vi "Get_Ch_data_from_file.vi"(0 "Filename":path, 9 "Channel names":string[](array[string]), 11 "Start of read offset (chars.: 0)":i32, 12 "Averaging Time(s)":dbl=5.0) -> (4 "exists?":bool, 6 "File Channels":string[](array[string]), 10 "Times":dbl[](array[numeric]) format="%.2f", 15 "Ch Data":dbl[][](array[numeric]) format="%.2f")   [LabVIEW 2010]
uses:
  <vilib>/Analysis/NI_AALBase.lvlib
panel:
  out "Time difference":dbl format="%.2f"
  in  "stop":bool
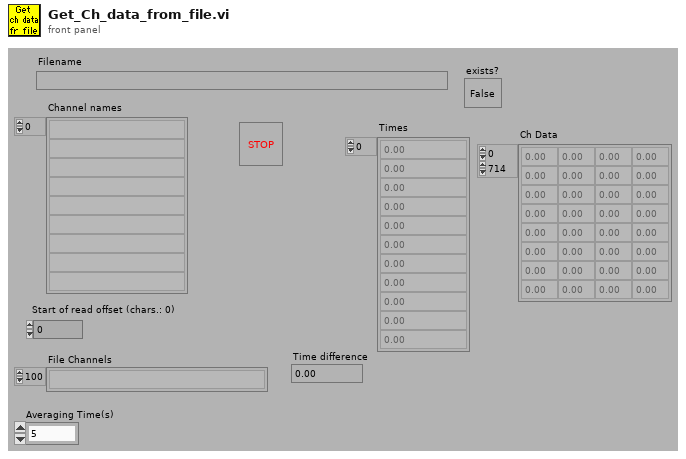
[diagram p1: front panel]
types:
  T1 = cluster{"second":i32, "minute":i32, "hour":i32, "day of month":i32, "month":i32, "year":i32, "day of week":i32, "day of year":i32, "is DST":i32}
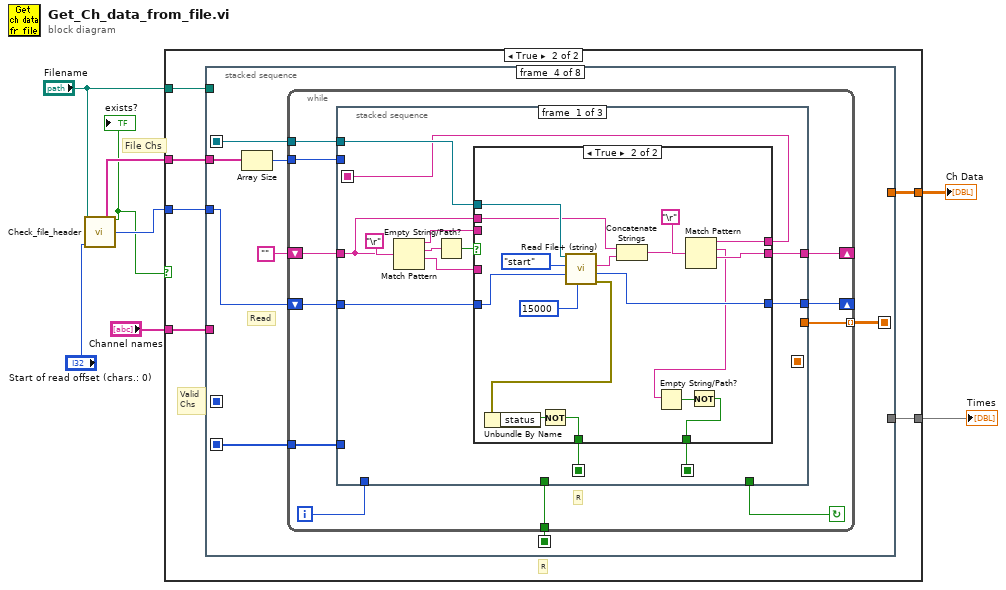
[diagram p0: block diagram]
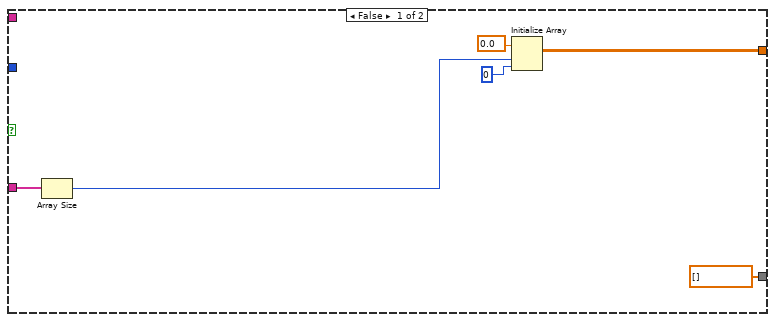
[diagram p2: hidden frame]
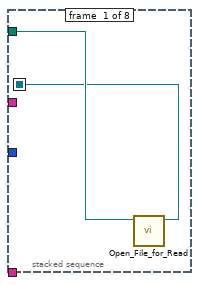
[diagram p3: hidden frame]
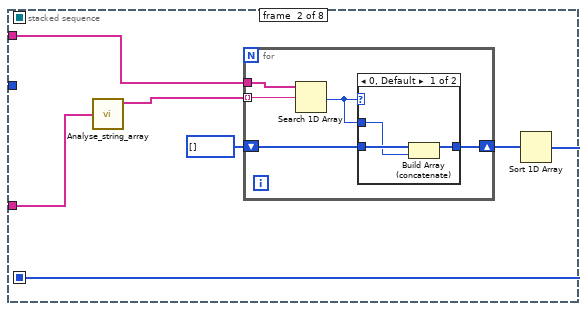
[diagram p4: hidden frame]
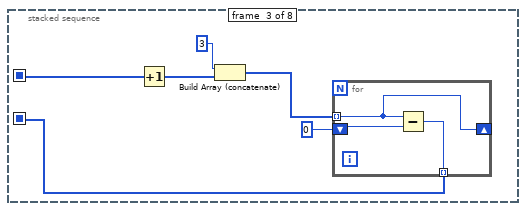
[diagram p6: hidden frame]
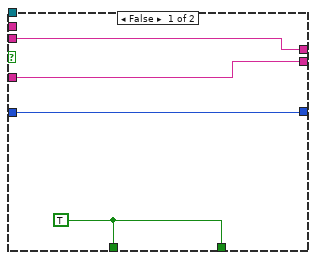
[diagram p7: hidden frame]
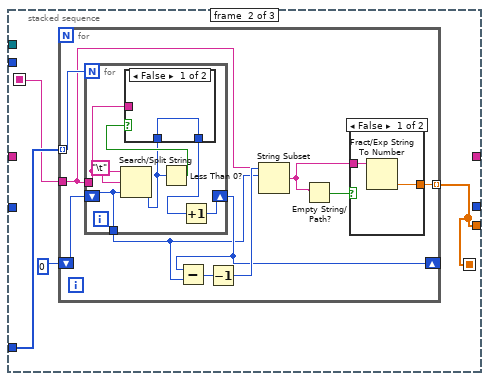
[diagram p8: hidden frame]
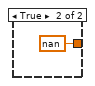
[diagram p9: hidden frame]
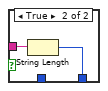
[diagram p10: hidden frame]
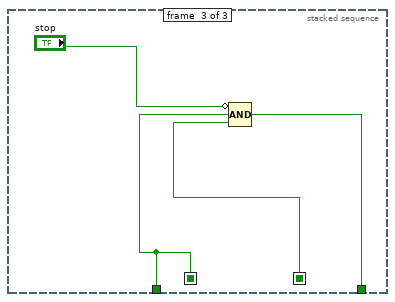
[diagram p11: hidden frame]
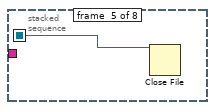
[diagram p12: hidden frame]
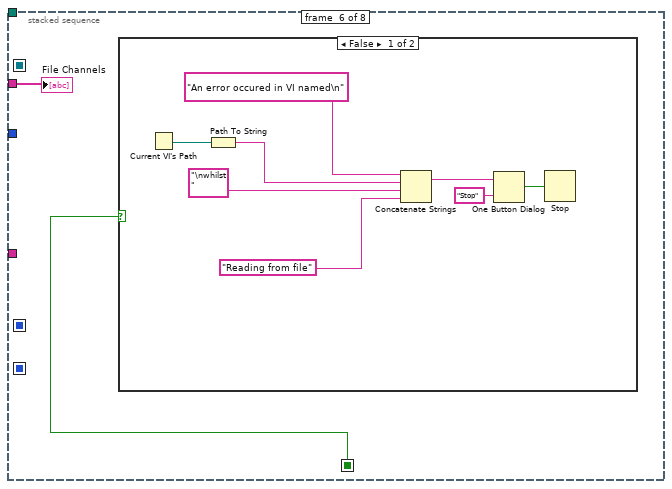
[diagram p13: hidden frame]
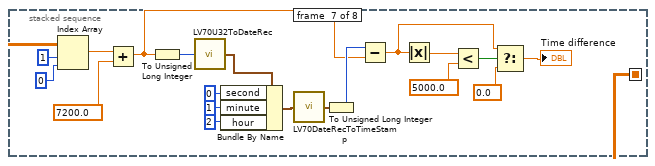
[diagram p15: hidden frame]
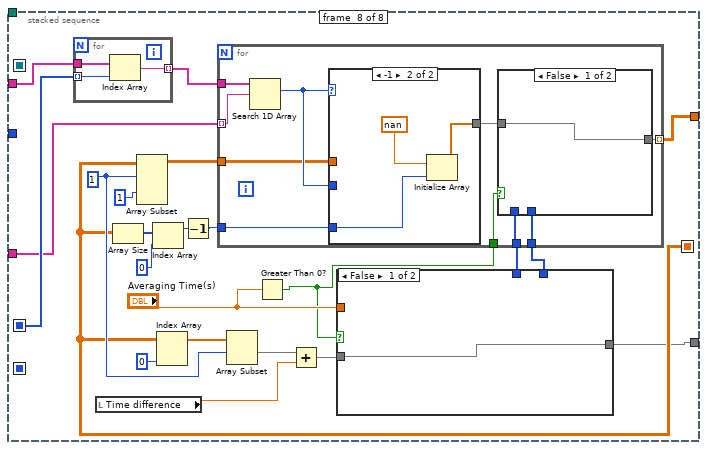
[diagram p16: hidden frame]
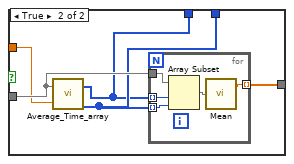
[diagram p17: hidden frame]
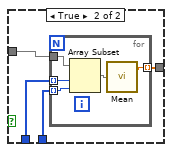
[diagram p18: hidden frame]
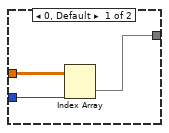
[diagram p19: hidden frame]
diagram:
  # "File Chs"
  n1 = call "Check_file_header.vi"("Filename"="Filename", "Start of read offset (chars.: 0)"="Start of read offset (chars.: 0)") -> ("File Channels"=w7:string[], "exists?"=w4:bool, "Start of data (bytes)"=w8:i32)  [unwired: 2 in, 9 out]
  "exists?" <- w4
  n2 = case shown="True" w4 {
    tunnel: w8 -> [_ w19]
    tunnel: w7 -> [_ w18]
    tunnel: "Filename" -> [_ w20]
    tunnel: [w9 w16] -> w3
    tunnel: [dbl[] [] w15] -> w2
    tunnel: "Channel names" -> [w11 w17]
    frame False {
      n3 = Array Size(array=w11) -> (size(s)=w10:i32)
      n4 = Initialize Array(0.0, w10, 0 ("Dimension Size")) -> (w9:dbl[][])
    }
    frame True {
      # "Valid\nChs"
      # "R"
      n5 = stacked-sequence {
        seq-local: [w21 _ _ _ _ _ _ _] -> [_ _ _ w53 w131 _ _ _]
        seq-local: [_ _ _ w50 _ _ _ _] -> [_ _ _ _ _ w133 _ _]
        seq-local: [_ _ _ w48 _ _ _ _] -> [_ _ _ _ _ _ w159 w173]
        seq-local: [_ _ w41 _ _ _ _ _] -> [_ _ _ w47 _ _ _ _]
        seq-local: [_ w25 _ _ _ _ _ _] -> [_ _ w39 _ _ _ _ w178]
        tunnel: w20 -> [w22 _ _ _ _ _ _ _]
        tunnel: w19 -> [_ _ _ w52 _ _ _ _]
        tunnel: w18 -> [_ w28 _ w49 _ w132 _ w177]
        tunnel: w17 -> [_ w24 _ _ _ _ _ w176]
        tunnel: [_ _ _ _ _ _ _ w169] -> w16
        tunnel: [_ _ _ _ _ _ _ w166] -> w15
        frame #0 {
          n6 = call "Open_File_for_Read.vi"("file path"=w22) -> ("refnum"=w21:refnum<file>)  [unwired: 1 in, 9 out]
        }
        frame #1 {
          n7 = call "Analyse_string_array.vi"("String array"=w24) -> ("Unique strings"=w23:string[])  [unwired: 2 out]
          n8 = for {
            tunnel: w28 -> [w33]
            tunnel: w23 -> [w32] mode=indexing
            shift-right: [w30] -> w26
            shift-left: i32[] [] -> [w31]
            n9 = Search 1D Array(1D array=w33, element=w32) -> (index of element=w29:i32)  [unwired: 1 out]
            n10 = case shown="0, Default" w29 {
              tunnel: w31 -> [w36 w37]
              tunnel: [w34 w37] -> w30
              tunnel: w29 -> [w35 _]
              frame 0, Default {
                n11 = Build Array (concatenate)(w36, w35) -> (w34:i32[])
              }
              frame -1 {
              }
            }
          }
          n12 = Sort 1D Array(array=w26) -> (sorted array=w25:i32[])
        }
        frame #2 {
          n13 = Increment(x=w39) -> (x+1=w38:i32[])
          n14 = Build Array (concatenate)(3 ("t"), w38) -> (w40:i32[])
          n15 = for {
            shift-right: [w45] -> _
            shift-left: 0 -> [w46]
            tunnel: w40 -> [w45] mode=indexing
            tunnel: [w44] -> w41 mode=indexing
            n16 = Subtract(x=w45, y=w46) -> (x-y=w44:i32)
          }
        }
        frame #3 {
          # "Read"
          n17 = Array Size(array=w49) -> (size(s)=w51:i32)
          n18 = while {
            tunnel: w47 -> [w56]
            tunnel: [w58] -> w48 mode=indexing
            tunnel: [w59] -> w50
            tunnel: w51 -> [w60]
            tunnel: w53 -> [w62]
            shift-left: w52 -> [w64]
            shift-right: [w63] -> _
            shift-left: "" -> [w65]
            shift-right: [w61] -> _
            i -> [w57]
            stop <- w55 continue-if-true
            # "R"
            n19 = stacked-sequence {
              seq-local: [w67 _ _] -> [_ w101 _]
              seq-local: [w68 _ _] -> [_ _ w127]
              seq-local: [w69 _ _] -> [_ _ w128]
              seq-local: [_ w100 _] -> [_ _ _]
              tunnel: w65 -> [w72 _ _]
              tunnel: w64 -> [w75 _ _]
              tunnel: [w74 _ _] -> w63
              tunnel: w62 -> [w73 _ _]
              tunnel: [w71 _ _] -> w61
              tunnel: w60 -> [_ _ _]
              tunnel: [_ _ w129] -> w55
              tunnel: [_ _ w128] -> w59
              tunnel: [_ w100 _] -> w58
              tunnel: w57 -> [_ _ _]
              tunnel: w56 -> [_ w103 _]
              frame #0 {
                n20 = Match Pattern(string=w72, regular expression="\r") -> (before substring=w66:string, match substring=w77:string, after substring=w70:string)  [unwired: 2 out]
                n21 = Empty String/Path?(string/path=w77) -> (empty?=w76:bool)
                n22 = case shown="True" w76 {
                  tunnel: w75 -> [w82 w98]
                  tunnel: [w82 w96] -> w74
                  tunnel: w73 -> [_ w95]
                  tunnel: w72 -> [_ w93]
                  tunnel: [w81 w90] -> w71
                  tunnel: w70 -> [w81 _]
                  tunnel: [w80 w86] -> w69
                  tunnel: [w80 w84] -> w68
                  tunnel: [w79 w83] -> w67
                  tunnel: w66 -> [w79 _]
                  frame False {
                    w80 = TRUE
                  }
                  frame True {
                    n23 = call <vilib>:"Read File+ (string).vi"("count"=15000, "pos offset (bytes:0)"=w98, "pos mode (rel. to current:2)"=enum16{"start", "end", "current"}."start", "refnum"=w95) -> ("error out"=w88:errorcluster, "mark after read (bytes)"=w96:i32, "string"=w94:string)  [unwired: 1 in, 4 out]
                    n24 = Unbundle By Name(w88) -> ("status"=w87:bool)
                    n25 = Not(x=w87) -> (.not. x?=w86:bool)
                    n26 = Concatenate Strings(w93, w94) -> (w91:string)
                    n27 = Match Pattern(string=w91, regular expression="\r") -> (before substring=w83:string, match substring=w89:string, after substring=w90:string)  [unwired: 2 out]
                    n28 = Empty String/Path?(string/path=w89) -> (empty?=w85:bool)
                    n29 = Not(x=w85) -> (.not. x?=w84:bool)
                  }
                }
              }
              frame #1 {
                n30 = for {
                  tunnel: w103 -> [w113] mode=indexing
                  tunnel: [w111] -> w100 mode=indexing
                  shift-right: [w105] -> _
                  shift-left: 0 -> [w110]
                  tunnel: w101 -> [w106]
                  n31 = for {
                    N: w113 -> [_]
                    shift-right: [w121] -> w105
                    shift-left: w110 -> [w122]
                    tunnel: w106 -> [w119]
                    tunnel: [w122] -> w104
                    n32 = Search/Split String(string=w119, search string/char (-)="\t", offset (0)=w122) -> (offset of match=w117:i32)  [unwired: 2 out]
                    n33 = Less Than 0?(x=w117) -> (x < 0?=w120:bool)
                    n34 = case shown="False" w120 {
                      tunnel: w119 -> [_ w126]
                      tunnel: [w124 w125] -> w118
                      tunnel: w117 -> [w124 _]
                      frame False {
                      }
                      frame True {
                        n35 = String Length(string=w126) -> (length=w125:i32)
                      }
                    }
                    n36 = Increment(x=w118) -> (x+1=w121:i32)
                  }
                  n37 = Subtract(x=w105, y=w104) -> (x-y=w109:i32)
                  n38 = Decrement(x=w109) -> (x-1=w108:i32)
                  n39 = String Subset(string=w106, offset (0)=w104, length (rest)=w108) -> (substring=w107:string)
                  n40 = Empty String/Path?(string/path=w107) -> (empty?=w112:bool)
                  n41 = case shown="False" w112 {
                    tunnel: w107 -> [w115 _]
                    tunnel: [w114 nan] -> w111
                    frame False {
                      n42 = Fract/Exp String To Number(string=w115) -> (number=w114:dbl)  [unwired: 4 out]
                    }
                    frame True {
                    }
                  }
                }
              }
              frame #2 {
                n43 = Compound Arithmetic op=AND(invert "stop", w128, w127) -> (w129:bool)
              }
            }
          }
        }
        frame #4 {
          n44 = Close File(refnum=w131) -> ()  [unwired: 1 in, 2 out]
        }
        frame #5 {
          n45 = case shown="False" w133 {
            frame False {
              n46 = Current VI's Path() -> (path=w134:path)
              n47 = Path To String(path=w134) -> (string=w140:string)
              n48 = Concatenate Strings("An error occured in VI named\n", w140, "\nwhilst ", "Reading from file") -> (w138:string)
              n49 = One Button Dialog(message=w138, button name ("OK")="Stop") -> (true=w136:bool)
              n50 = Stop(stop? (T)=w136) -> ()
            }
            frame True {
            }
          }
          "File Channels" <- w132
        }
        frame #6 {
          n51 = Index Array(array=w159, index (row)=1 ("Index"), index (col)=0 ("Index")) -> (element=w146:dbl)
          n52 = Add(x=w146, y=7200.0) -> (x+y=w143:dbl)
          n53 = To Unsigned Long Integer(number=w143) -> (unsigned 32bit integer=w153:u32)
          n54 = call <vilib>:"LV70U32ToDateRec.vi"("Time"=w153) -> ("date time rec"=w158:T1)
          n55 = Bundle By Name(cluster=w158, "second"=0 ("Bundle Element"), "minute"=1 ("Bundle Element"), "hour"=2 ("Bundle Element")) -> (w154:T1)
          n56 = call <vilib>:"LV70DateRecToTimeStamp.vi"("date time rec"=w154) -> ("Time Stamp"=w142:timestamp)
          n57 = To Unsigned Long Integer(number=w142) -> (unsigned 32bit integer=w144:u32)
          n58 = Subtract(x=w144, y=w143) -> (x-y=w148:dbl)
          n59 = Absolute Value(x=w148) -> (abs(x)=w152:dbl)
          n60 = Less?(x=w152, y=5000.0) -> (x < y?=w150:bool)
          n61 = Select(t=w148, s=w150, f=0.0) -> (s? t:f=→"Time difference":dbl)
        }
        frame #7 {
          w181 = 1
          n62 = for {
            tunnel: w178 -> [w198] mode=indexing
            tunnel: w177 -> [w197]
            tunnel: [w196] -> w175 mode=indexing
            n63 = Index Array(array=w197, index=w198) -> (element=w196:string)
          }
          n64 = local read "Time difference"() -> (w179:dbl)
          n65 = Array Size(array=w173) -> (size(s)=w172:i32[])
          n66 = Array Subset(array=w173, index (row)=w181, index (col)=1) -> (w174:dbl[][])  [unwired: 2 in]
          n67 = Index Array(array=w172, index=0 ("Index")) -> (element=w170:i32)
          n68 = Index Array(array=w173, index (col)=0) -> (element=w182:dbl[])  [unwired: 1 in]
          n69 = Decrement(x=w170) -> (x-1=w168:i32)
          n70 = Array Subset(array=w182, index=w181) -> (w180:dbl[])  [unwired: 1 in]
          n71 = Greater Than 0?(x="Averaging Time(s)") -> (x > 0?=w162:bool)
          n72 = Add(x=w180, y=w179) -> (x+y=w167:dbl[])
          n73 = case shown="False" w162 {
            tunnel: w167 -> [w185 w190]
            tunnel: [w185 w189] -> w166
            tunnel: [_ w186] -> w165
            tunnel: [_ w188] -> w164
            tunnel: "Averaging Time(s)" -> [_ w187]
            frame False {
            }
            frame True {
              n74 = call "Average_Time_array.vi"("Average TIme (seconds)"=w187, "Centre Time in Seconds"=w190) -> ("Length"=w188:i32[], "Start"=w186:i32[])
              n75 = for {
                tunnel: w190 -> [w195]
                tunnel: w186 -> [w194] mode=indexing
                tunnel: w188 -> [w193] mode=indexing
                tunnel: [w191] -> w189 mode=indexing
                n76 = Array Subset(array=w195, index=w194, length=w193) -> (w192:dbl[])
                n77 = call <vilib>:"Mean.vi"("X"=w192) -> ("mean"=w191:dbl)  [unwired: 1 out]
              }
            }
          }
          n78 = for {
            tunnel: w176 -> [w208] mode=indexing
            tunnel: w175 -> [w207]
            tunnel: w174 -> [w205]
            tunnel: [w200] -> w169 mode=indexing
            tunnel: w168 -> [w204]
            tunnel: w165 -> [w202]
            tunnel: w164 -> [w201]
            tunnel: w162 -> [w199]
            n79 = Search 1D Array(1D array=w207, element=w208) -> (index of element=w206:i32)  [unwired: 1 out]
            n80 = case shown="-1" w206 {
              tunnel: w206 -> [w219 _]
              tunnel: w205 -> [w221 _]
              tunnel: [w220 w223] -> w203
              tunnel: w204 -> [_ w222]
              frame 0, Default {
                n81 = Index Array(array=w221, index (col)=w219) -> (element=w220:dbl[])  [unwired: 1 in]
              }
              frame -1 {
                n82 = Initialize Array(nan ("Number"), w222) -> (w223:dbl[])
              }
            }
            n83 = case shown="False" w199 {
              tunnel: w203 -> [w209 w213]
              tunnel: w202 -> [_ w212]
              tunnel: w201 -> [_ w211]
              tunnel: [w209 w210] -> w200
              frame False {
              }
              frame True {
                n84 = for {
                  tunnel: w213 -> [w218]
                  tunnel: w212 -> [w217] mode=indexing
                  tunnel: w211 -> [w216] mode=indexing
                  tunnel: [w214] -> w210 mode=indexing
                  n85 = Array Subset(array=w218, index=w217, length=w216) -> (w215:dbl[])
                  n86 = call <vilib>:"Mean.vi"("X"=w215) -> ("mean"=w214:dbl)  [unwired: 1 out]
                }
              }
            }
          }
        }
      }
    }
  }
  "Ch Data" <- w3
  "Times" <- w2
